vi "Global FTT Data.vi"(8 "error in (no error)":errorcluster, 10 "Mode":enum16{"Read", "Write"}(ring), 11 "Display":T2) -> (0 "error out":errorcluster, 3 "Cluster":T2)   [LabVIEW 2014]
uses:
  Type'def/FTT Display Type.ctl
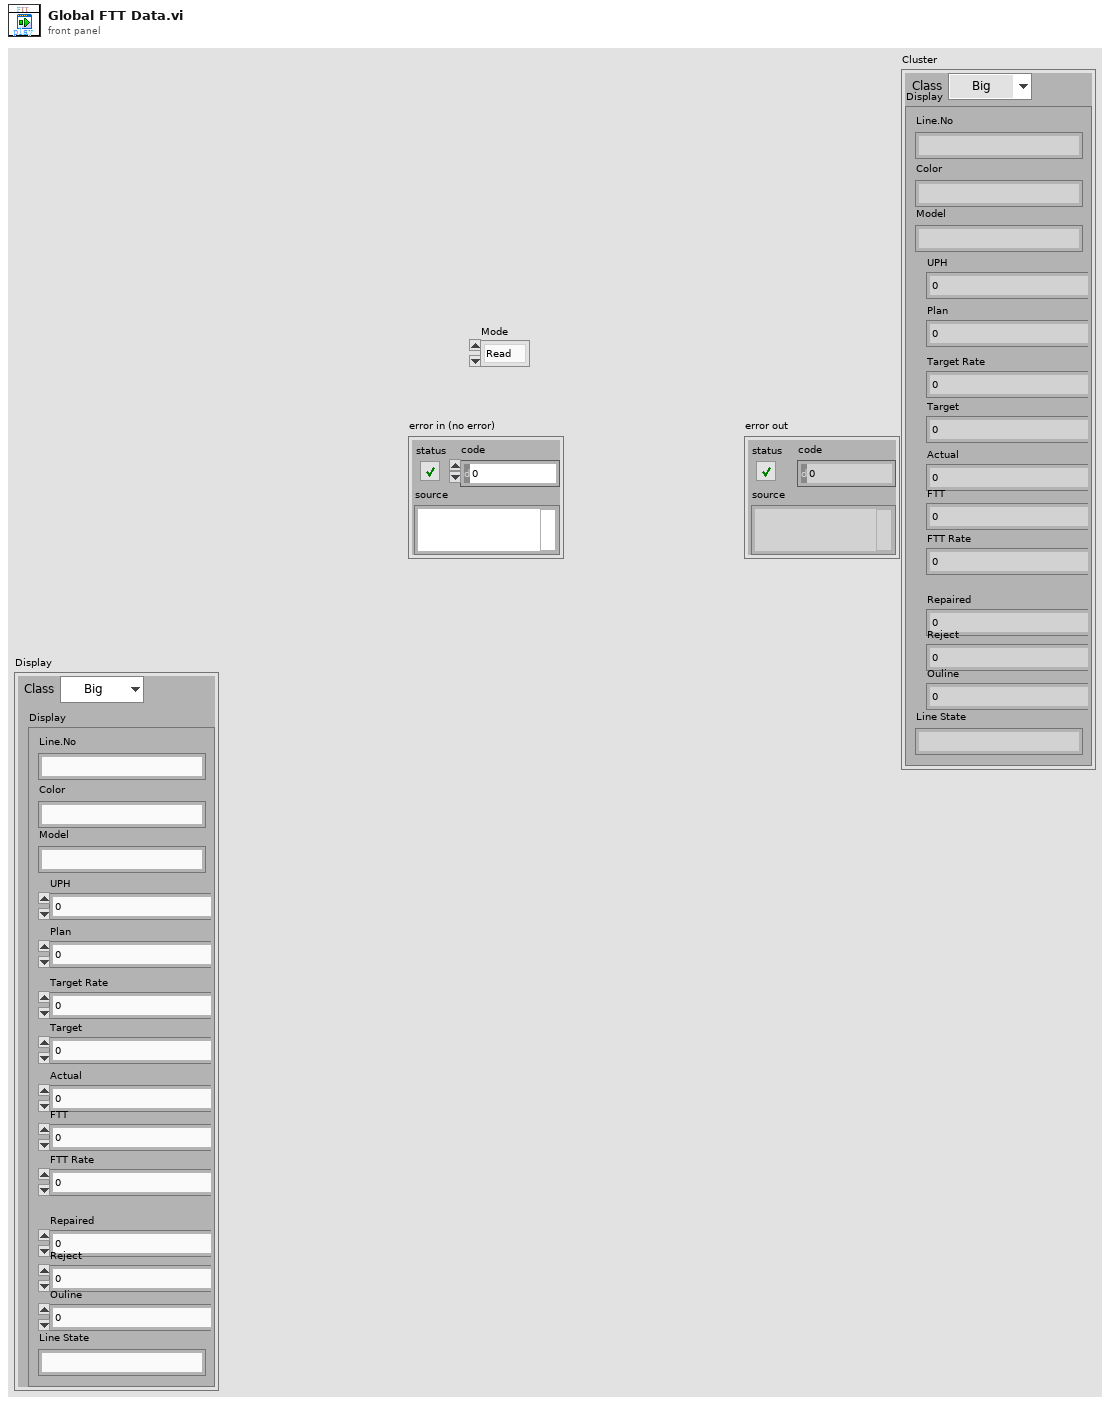
[diagram p1: front panel]
types:
  T1 = typedef "FTT Display Type.ctl" = cluster{"Line.No":string, "Model":string, "Color":string, "UPH":dbl, "Plan":dbl, "Target Rate":dbl, "Target ":dbl, "Actual":dbl, "FTT":dbl, "FTT Rate":dbl, "Repaired":dbl, "Reject":dbl, "Ouline":dbl, "Line State":string}
  T2 = cluster{"Display":T1, "Class":enum16{"Big", "Small"}}
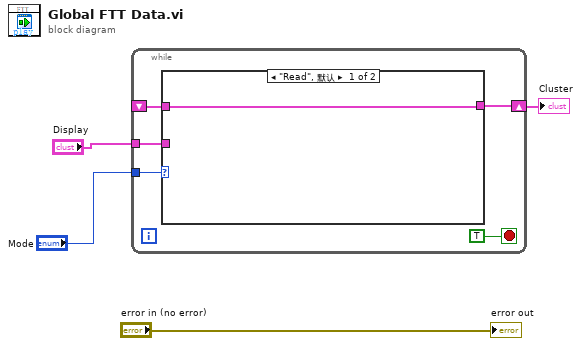
[diagram p0: block diagram]
diagram:
  n1 = while {
    tunnel: "Mode" -> [w8]
    tunnel: "Display" -> [w7]
    shift-right: [w6] -> w2
    shift-left: _ -> [w5]
    stop <- TRUE stop-if-true
    n2 = case shown="\"Read\", 默认" w8 {
      tunnel: w7 -> [_ w11]
      tunnel: [w10 w11] -> w6
      tunnel: w5 -> [w10 _]
      frame "Read", Default {
      }
      frame "Write" {
      }
    }
  }
  "Cluster" <- w2
  "error out" <- "error in (no error)"
